vi "IMAQ LL-Sequence.vi"(7 "Skip table":i32[](array[numeric]), 8 "ErrIn":errorcluster, 11 "IF Name":string="img0") -> (0 "ErrOut":errorcluster, 3 "ImgOut":T1[](array[typedef]))   [LabVIEW 2013]
doc: "Use this template to build a VI to use as a subVI."
uses:
  <vilib>/vision/Image Controls.llb/IMAQ Image.ctl
panel:
  in  "Number of images":i32=10
  # "Input Parameters"
  # "Output Parameters"
  # "VI Description:\nLow Level IMAQ Sequence"
  # ":: MVI Framework V1.0 ::\nAuthor:Gaoke Yang\nEmail: gaoke.yang@yahoo.com\nWeb: www.mvicontrol.com\nCopyright (C) 2013, MVI Technologies All Rights Reserved"
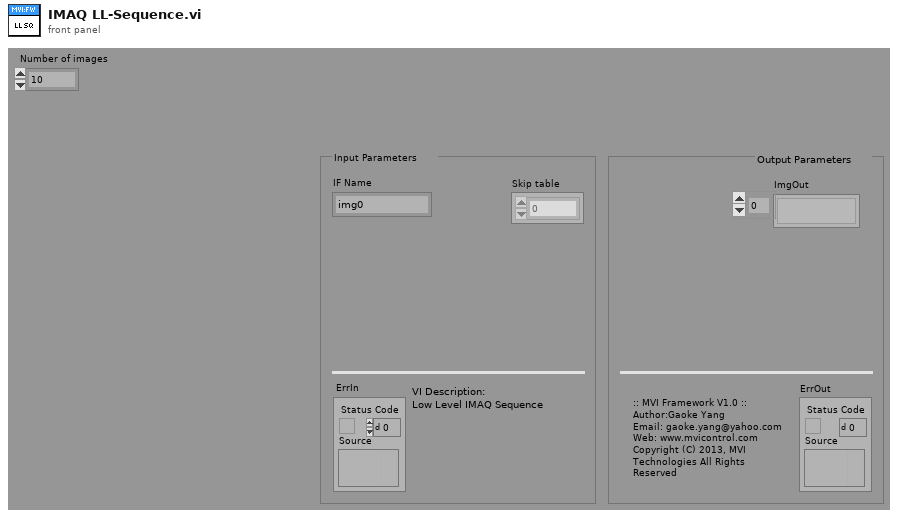
[diagram p1: front panel]
types:
  T1 = typedef "IMAQ Image.ctl" = refnum<image>
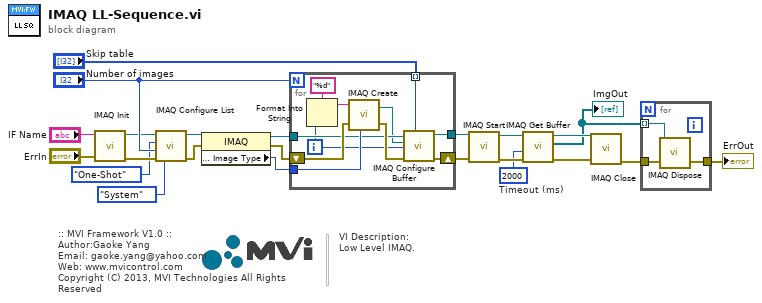
[diagram p0: block diagram]
diagram:
  w13 = 2000  # Timeout (ms)
  # "VI Description:\nLow Level IMAQ."
  # ":: MVI Framework V1.0 ::\nAuthor:Gaoke Yang\nEmail: gaoke.yang@yahoo.com\nWeb: www.mvicontrol.com\nCopyright (C) 2013, MVI Technologies All Rights Reserved"
  n1 = call <vilib>:"IMAQ Init.vi"("error in (no error)"="ErrIn", "Interface Name"="IF Name") -> ("error out"=w7:errorcluster, "IMAQ Session Out"=w8:refnum<k11>)  [unwired: 8 out]
  n2 = call <vilib>:"IMAQ Configure List.vi"("Memory Location"=enum16{"System", "Onboard"}."System", "error in (no error)"=w7, "Number of buffers"="Number of images", "Continuous?"=enum16{"One-Shot", "Continuous"}."One-Shot" ("Continuous ?"), "IMAQ Session In"=w8) -> ("error out"=w4:errorcluster, "IMAQ Session Out"=w5:refnum<k11>)  [unwired: 1 in, 4 out]
  n3 = property class="IMAQ"(reference=w5, error in=w4) -> (reference out=w10:refnum<k11>, error out=w12:errorcluster, "Image Parameters : Image Type"=w11:u32)
  n4 = for {
    N: "Number of images" -> [_]
    tunnel: w10 -> [w27]
    tunnel: w11 -> [w34]
    shift-right: [w29] -> w3
    shift-left: w12 -> [w33]
    tunnel: [w28] -> w2
    tunnel: "Skip table" -> [w24] mode=indexing
    i -> [w25]
    n5 = Format Into String(format string="%d", w25) -> (resulting string=w32:string)  [unwired: 2 in, 1 out]
    n6 = call "IMAQ Create"("Image Name"=w32, "Image Type"=w34, "error in (no error)"=w33) -> ("New Image"=w26:T1, "error out"=w30:errorcluster)  [unwired: 1 in, 1 out]
    n7 = call <vilib>:"IMAQ Configure Buffer.vi"("Skip Count"=w24, "error in (no error)"=w30, "Buffer Number"=w25, "Image In"=w26, "IMAQ Session In"=w27) -> ("error out"=w29:errorcluster, "IMAQ Session Out"=w28:refnum<k11>)  [unwired: 1 in, 4 out]
  }
  n8 = call <vilib>:"IMAQ Start.vi"("error in (no error)"=w3, "IMAQ Session In"=w2) -> ("error out"=w14:errorcluster, "IMAQ Session Out"=w15:refnum<k11>)  [unwired: 8 out]
  n9 = call <vilib>:"IMAQ Get Buffer.vi"("error in (no error)"=w14, "Timeout (ms)"=w13, "IMAQ Session In"=w15) -> ("error out"=w18:errorcluster, "Images Out"=w16:T1[], "IMAQ Session Out"=w17:refnum<k11>)  [unwired: 1 in, 5 out]
  "ImgOut" <- w16
  n10 = call <vilib>:"IMAQ Close.vi"("error in (no error)"=w18, "IMAQ Session In"=w17) -> ("error out"=w19:errorcluster)  [unwired: 9 out]
  n11 = for {
    tunnel: w19 -> [w36]
    tunnel: w16 -> [w37] mode=indexing
    tunnel: [w35] -> w20
    n12 = call "IMAQ Dispose"("Image"=w37, "error in (no error)"=w36) -> ("error out"=w35:errorcluster)  [unwired: 1 in, 3 out]
  }
  "ErrOut" <- w20
